vi "VIPM Uninstall All VI Packages By Name.vi"   [LabVIEW 2016, in "Script.lvlib"]
uses:
  Script.lvlib
  <vilib>/Wiresmith Technology/G CLI/Argument Parser/Option Class/Option Configuration.ctl
  <vilib>/Wiresmith Technology/G CLI/Argument Parser/Option Class/Argument Type.ctl
  <vilib>/Wiresmith Technology/G CLI/CLI Class/CLI.lvclass
  <vilib>/Wiresmith Technology/G CLI/Argument Parser/Option Class/Option.lvclass
  <vilib>/Wiresmith Technology/G CLI/Argument Parser/Option Set Class/Option Set.lvclass
  <vilib>/JKI/VIPM API/VIPM API_vipm_api.lvlib
types:
  T1 = typedef "Option Parser.lvlib/Option.lvclass/Option Configuration.ctl" = cluster{"Option Type":T2, "Option Labels":string[], "Key":string, "Description":string, "Required":bool, "Default Value":string}
  T2 = typedef "Option Parser.lvlib/Option.lvclass/Argument Type.ctl" = enum16{"flag", "value"}
  T3 = typedef "VIPM API_vipm_api.lvlib/Library Contents Cluster_vipm_api.ctl" = cluster{"Package Name":string, "Version":string, "Display Name":string, "Repository Name":string, "Company Name":string, "License Type":string, "Installed":bool, "Deprecated":bool, "Dependency or Conflict Problem":bool, "Downloaded":bool}
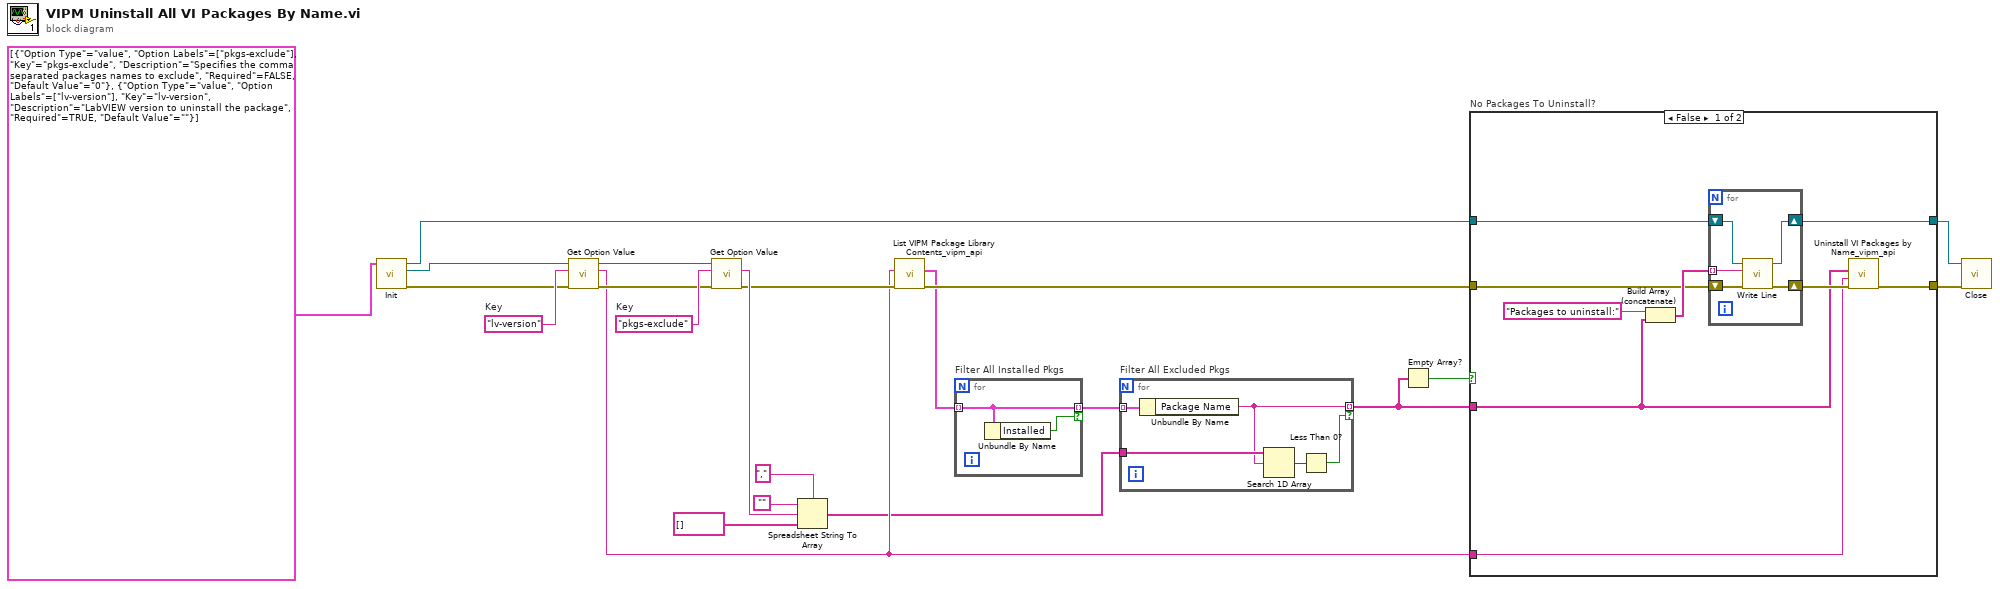
[diagram p0: block diagram]
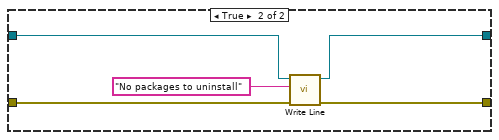
[diagram p2: hidden frame]
diagram:
  w17 = "lv-version"  # Key
  w22 = "pkgs-exclude"  # Key
  n1 = call "Init.vi"("Options"=T1[] [{"Option Type"=enum."value", "Option Labels"=["pkgs-exclude"], "Key"="pkgs-exclude", "Description"="Specifies the comma separated packages names to exclude", "Required"=FALSE, "Default Value"="0"}, {"Option Type"=enum."value", "Option Labels"=["lv-version"], "Key"="lv-version", "Description"="LabVIEW version to uninstall the package", "Required"=TRUE, "Default Value"=""}]) -> ("error out"=w12:errorcluster, "Option Set out"=w11:refnum<class "Option Set.lvclass">, "CLI out"=w10:refnum<class "CLI.lvclass">)  [unwired: 8 in]
  n2 = call <vilib>:"Get Option Value.vi"("error in (no error)"=w12, "Option Key"=w17, "Option Set in"=w11) -> ("error out"=w16:errorcluster, "Value"=w6:string, "Option Set out"=w15:refnum<class "Option Set.lvclass">)  [unwired: 5 in, 1 out]
  n3 = call <vilib>:"Get Option Value.vi"("error in (no error)"=w16, "Option Key"=w22, "Option Set in"=w15) -> ("error out"=w8:errorcluster, "Value"=w14:string)  [unwired: 5 in, 2 out]
  n4 = Spreadsheet String To Array(delimiter (Tab)=",", format string="", spreadsheet string=w14, array type (2D Dbl)=string[] [] ("Value")) -> (array=w3:string[])
  n5 = call <vilib>:"List VIPM Package Library Contents_vipm_api.vi"("error in (no error)"=w8, "LabVIEW Version"=w6) -> ("error out"=w7:errorcluster, "Library Contents []"=w5:T3[])  [unwired: 7 in, 1 out]
  n6 = for "Filter All Installed Pkgs" {
    tunnel: w5 -> [w24] mode=indexing
    tunnel: [w24] -> w4 mode=indexing if=w23
    n7 = Unbundle By Name(w24) -> ("Installed"=w23:bool)
  }
  n8 = for "Filter All Excluded Pkgs" {
    tunnel: w4 -> [w29] mode=indexing
    tunnel: [w25] -> w2 mode=indexing if=w26
    tunnel: w3 -> [w28]
    n9 = Unbundle By Name(w29) -> ("Package Name"=w25:string)
    n10 = Search 1D Array(1D array=w28, element=w25) -> (index of element=w27:i32)  [unwired: 1 in]
    n11 = Less Than 0?(x=w27) -> (x < 0?=w26:bool)
  }
  n12 = Empty Array?(array=w2) -> (empty?=w1:bool)
  n13 = case "No Packages To Uninstall?" shown="False" w1 {
    tunnel: [w37 w48] -> w21
    tunnel: [w36 w47] -> w20
    tunnel: w10 -> [w33 w46]
    tunnel: w7 -> [w32 w45]
    tunnel: w6 -> [w31 _]
    tunnel: w2 -> [w30 _]
    frame False {
      n14 = Build Array (concatenate)("Packages to uninstall:" ("delimiter (Tab)"), w30) -> (w34:string[])
      n15 = for {
        shift-right: [w41] -> w36
        shift-left: w33 -> [w43]
        shift-right: [w42] -> w38
        shift-left: w32 -> [w40]
        tunnel: w34 -> [w39] mode=indexing
        n16 = call <vilib>:"Write Line.vi"("error in (no error)"=w40, "Text to Write"=w39, "CLI in"=w43) -> ("error out"=w42:errorcluster, "CLI out"=w41:refnum<class "CLI.lvclass">)  [unwired: 7 in]
      }
      n17 = call <vilib>:"Uninstall VI Packages by Name_vipm_api.vi"("error in (no error)"=w38, "LabVIEW Version"=w31, "Package Names to Uninstall []"=w30) -> ("error out"=w37:errorcluster)  [unwired: 8 in]
    }
    frame True {
      n18 = call <vilib>:"Write Line.vi"("error in (no error)"=w45, "Text to Write"="No packages to uninstall" ("delimiter (Tab)"), "CLI in"=w46) -> ("error out"=w48:errorcluster, "CLI out"=w47:refnum<class "CLI.lvclass">)  [unwired: 7 in]
    }
  }
  n19 = call "Close.vi"("error in (no error)"=w21, "CLI in"=w20) -> ()  [unwired: 10 in]
